vi "отчет по плавке1.vi"(8 "disk":string, 11 "rasp":string[][](array[string])) -> ()   [LabVIEW 2016]
uses:
  Granule-2000AT/PC/llb/Library.lvlib
panel:
  out "P plasmatron":string[](array[string])
  out "P camera":string[](array[string])
  out "PV":string[](array[string])
  out "U_ist":string[](array[string])
  out "I_ist":string[](array[string])
  out "Actual speed":string[](array[string])
  out "Rotation":string[](array[string])
  out "data":string[](array[string])
  out "Mark":string
  out "Billet numer":string caption="Billet\nnumer"
  out "End record":string caption="End of\nrecord"
  out "Start record":string caption="Start\nrecording"
  out "Diametr":string
  in  "Tab Control":T1(tab)
  out "Rotation":cluster{"data dbl":dbl[], dbl[]}(graph)
  out "Actual sped":cluster{"data dbl":dbl[], dbl[]}(graph)
  out "PV зазор":cluster{"data dbl":dbl[], dbl[]}(graph)
  out "I_ист":cluster{"data dbl":dbl[], dbl[]}(graph)
  out "U_ист":cluster{"data dbl":dbl[], dbl[]}(graph)
  out "Presure":cluster{"data dbl":dbl[], dbl[]}[](graph)
  out "Status":u8(slide) scale=0.0..3.0
  in  "Process Stop Button":bool
  in  "Copy Button":bool
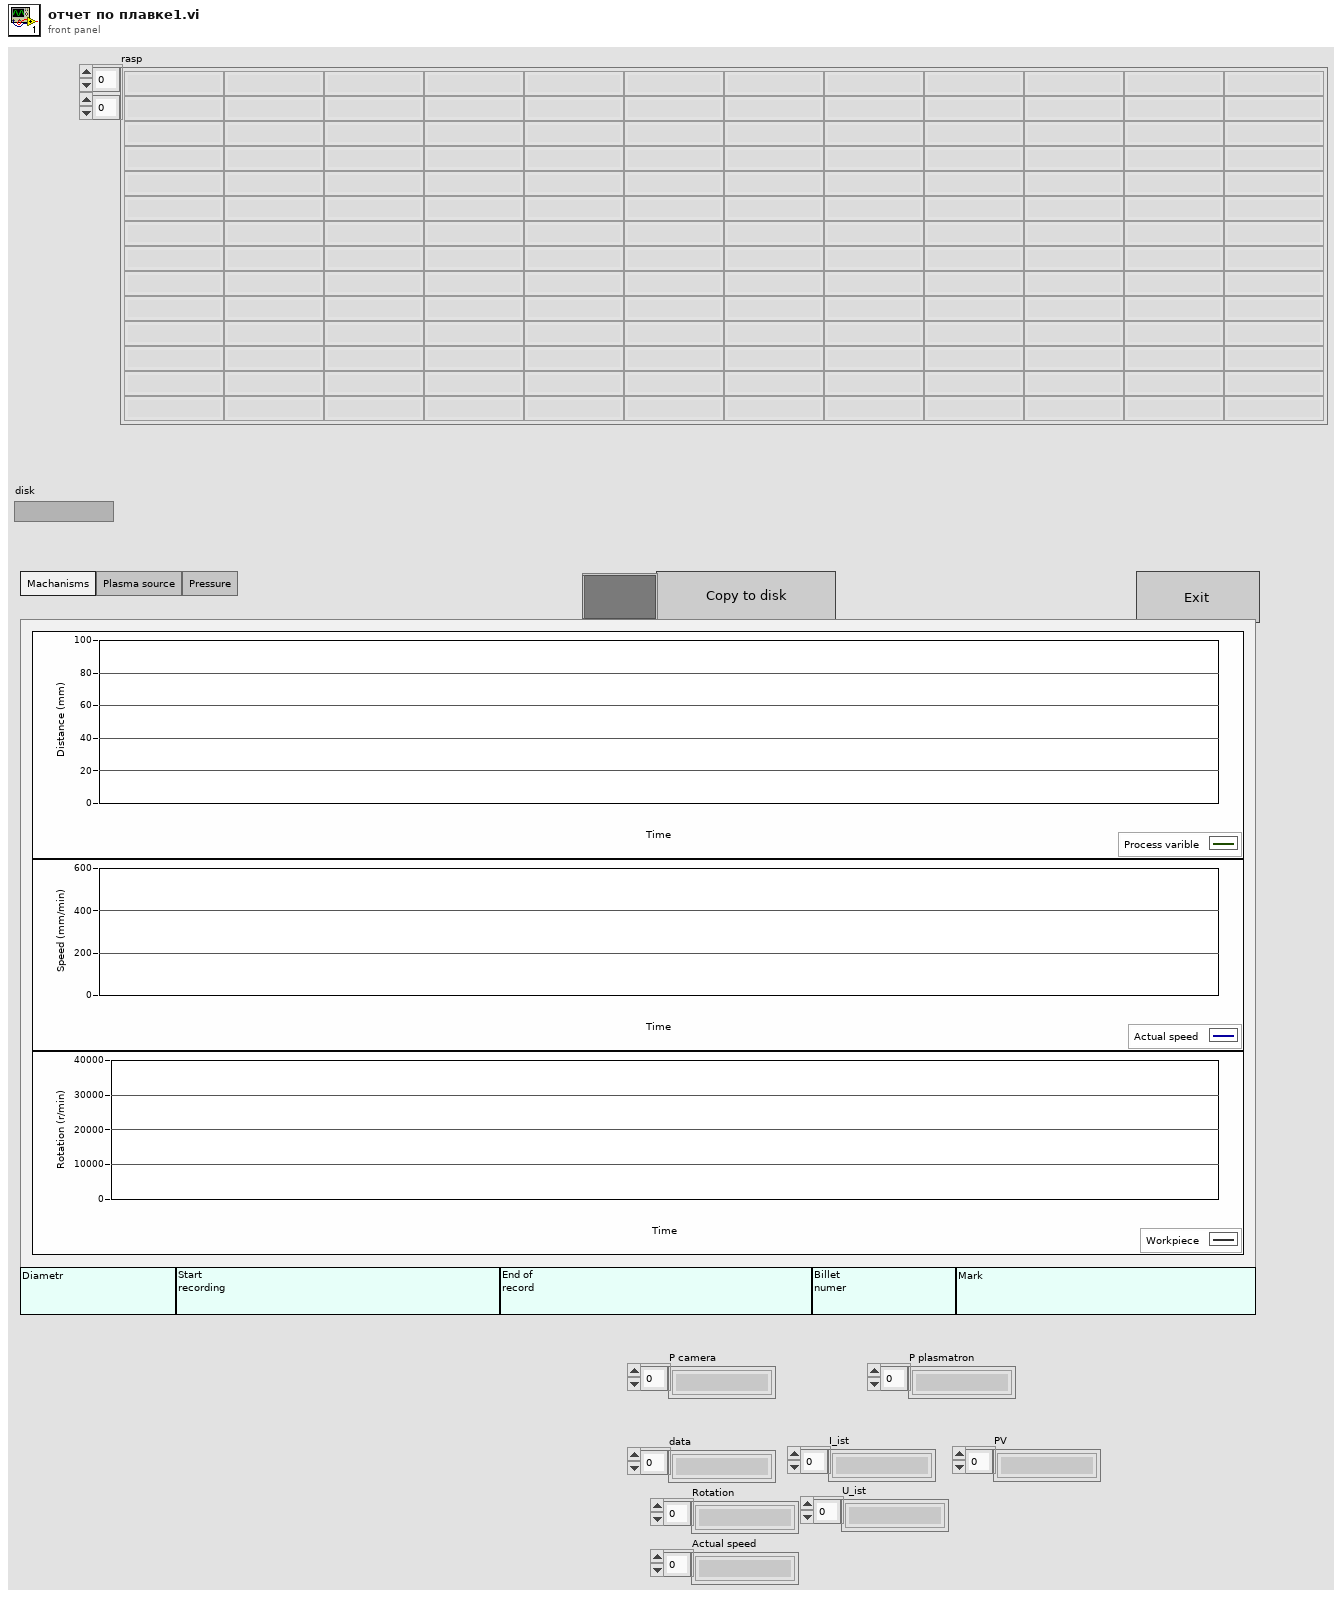
[diagram p1: front panel]
types:
  T1 = enum32{"Machanisms", "Plasma source", "Pressure"}
  T2 = cluster{cluster{"data dbl":dbl[], dbl[]}, cluster{"data dbl":dbl[], dbl[]}, cluster{"data dbl":dbl[], dbl[]}, "String":string, "String":string, "String":string, "String":string, "String":string}
  T3 = cluster{"String":string, "String":string, "String":string, "String":string, "String":string, cluster{"data dbl":dbl[], dbl[]}, cluster{"data dbl":dbl[], dbl[]}, cluster{"data dbl":dbl[], dbl[]}[]}
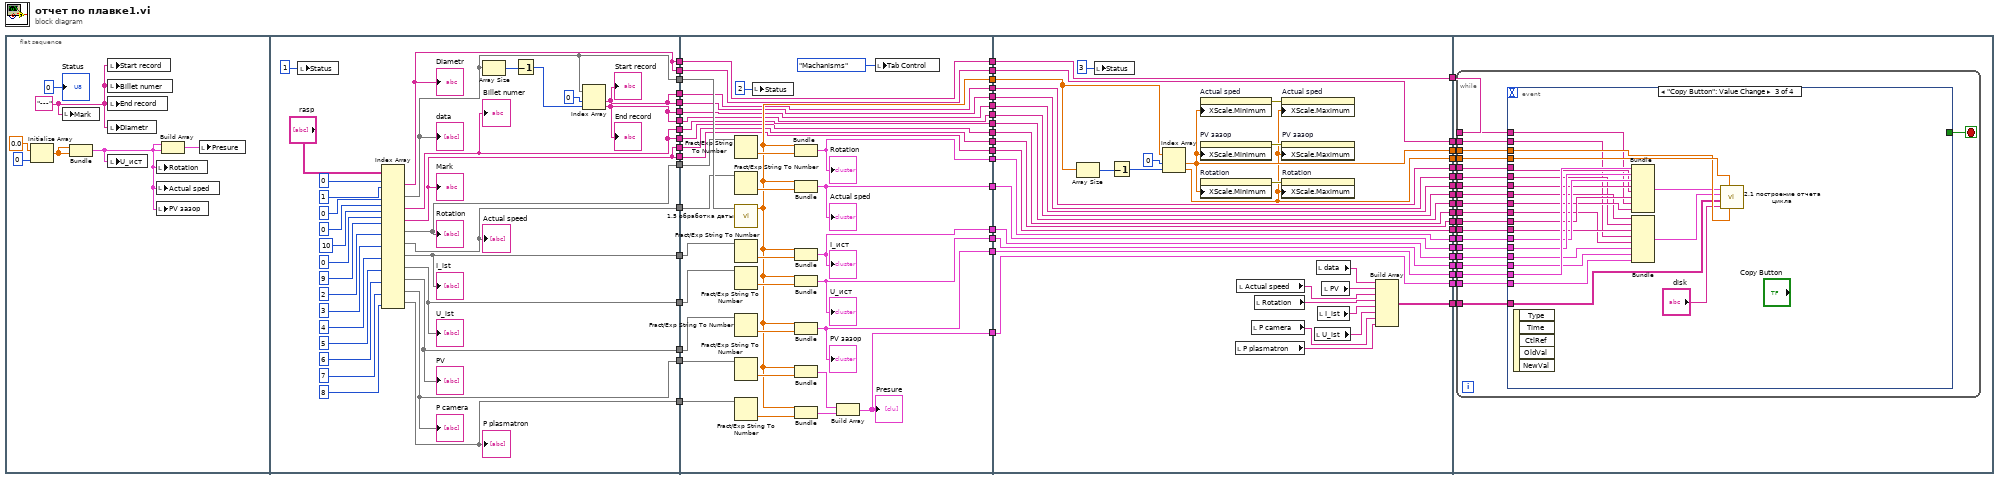
[diagram p0: block diagram]
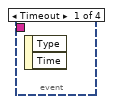
[diagram p2: hidden frame]
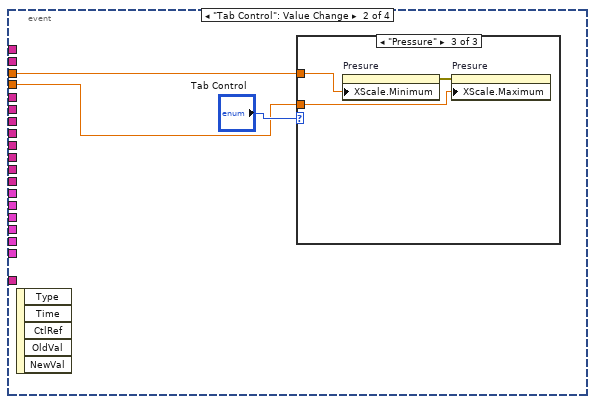
[diagram p3: hidden frame]
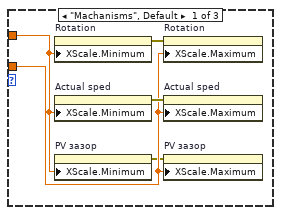
[diagram p4: hidden frame]
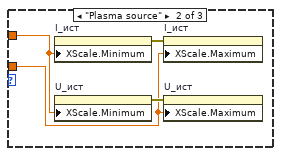
[diagram p5: hidden frame]
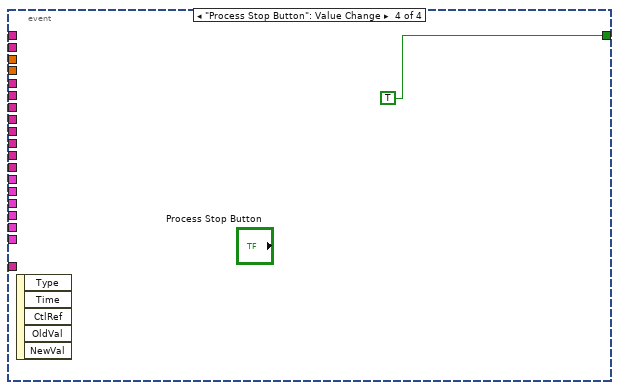
[diagram p6: hidden frame]
diagram:
  n1 = flat-sequence {
    tunnel: [w83] -> w54
    tunnel: [w81] -> w53
    tunnel: [w79] -> w52
    tunnel: [w75] -> w51
    tunnel: [w74] -> w50
    tunnel: [w73] -> w49
    tunnel: [w70] -> w48
    tunnel: [w69] -> w47
    tunnel: [w67] -> w34
    tunnel: [w66] -> w31
    tunnel: [w65] -> w28
    tunnel: [w64] -> w25
    tunnel: [w63] -> w22
    tunnel: [w67] -> w19
    tunnel: [w66] -> w16
    tunnel: [w65] -> w13
    tunnel: [w64] -> w10
    tunnel: [w63] -> w7
    tunnel: w54 -> [w129]
    tunnel: w53 -> [w128]
    tunnel: w52 -> [w126]
    tunnel: w51 -> [w124]
    tunnel: w50 -> [w122]
    tunnel: w49 -> [w119]
    tunnel: w48 -> [w116]
    tunnel: w47 -> [w115]
    tunnel: [w111] -> w46
    tunnel: [w109] -> w41
    tunnel: [w108] -> w39
    tunnel: [w107] -> w37
    tunnel: [w106] -> w35
    tunnel: w34 -> [w106]
    tunnel: [w105] -> w32
    tunnel: w31 -> [w105]
    tunnel: [w104] -> w29
    tunnel: w28 -> [w104]
    tunnel: [w103] -> w26
    tunnel: w25 -> [w103]
    tunnel: [w102] -> w23
    tunnel: w22 -> [w102]
    tunnel: [w101] -> w20
    tunnel: w19 -> [w101]
    tunnel: [w100] -> w17
    tunnel: w16 -> [w100]
    tunnel: [w99] -> w14
    tunnel: w13 -> [w99]
    tunnel: [w98] -> w11
    tunnel: w10 -> [w98]
    tunnel: [w97] -> w8
    tunnel: w7 -> [w97]
    tunnel: [w96] -> w5
    tunnel: [w95] -> w3
    tunnel: [w94] -> w1
    tunnel: w46 -> [w163]
    tunnel: [w157] -> w45
    tunnel: [w156] -> w44
    tunnel: [w146] -> w43
    tunnel: [w145] -> w42
    tunnel: w41 -> [w145]
    tunnel: [w144] -> w40
    tunnel: w39 -> [w144]
    tunnel: [w143] -> w38
    tunnel: w37 -> [w143]
    tunnel: [w142] -> w36
    tunnel: w35 -> [w142]
    tunnel: [w141] -> w33
    tunnel: w32 -> [w141]
    tunnel: [w140] -> w30
    tunnel: w29 -> [w140]
    tunnel: [w139] -> w27
    tunnel: w26 -> [w139]
    tunnel: [w138] -> w24
    tunnel: w23 -> [w138]
    tunnel: [w137] -> w21
    tunnel: w20 -> [w137]
    tunnel: [w136] -> w18
    tunnel: w17 -> [w136]
    tunnel: [w135] -> w15
    tunnel: w14 -> [w135]
    tunnel: [w134] -> w12
    tunnel: w11 -> [w134]
    tunnel: [w133] -> w9
    tunnel: w8 -> [w133]
    tunnel: [w132] -> w6
    tunnel: w5 -> [w132]
    tunnel: [w131] -> w4
    tunnel: w3 -> [w131]
    tunnel: [w130] -> w2
    tunnel: w1 -> [w130]
    tunnel: w45 -> [w183]
    tunnel: w44 -> [w182]
    tunnel: w43 -> [w181]
    tunnel: w42 -> [w180]
    tunnel: w40 -> [w179]
    tunnel: w38 -> [w178]
    tunnel: w36 -> [w177]
    tunnel: w33 -> [w176]
    tunnel: w30 -> [w175]
    tunnel: w27 -> [w174]
    tunnel: w24 -> [w173]
    tunnel: w21 -> [w172]
    tunnel: w18 -> [w171]
    tunnel: w15 -> [w170]
    tunnel: w12 -> [w169]
    tunnel: w9 -> [w168]
    tunnel: w6 -> [w167]
    tunnel: w4 -> [w166]
    tunnel: w2 -> [w165]
    frame #0 {
      w57 = "---" ("Billet numer")
      n2 = Initialize Array(0.0, 0 ("dimension size")) -> (w59:dbl[])
      n3 = local write "Mark"(w57) -> ()
      n4 = Bundle(w59, w59) -> (w56:cluster{dbl[], dbl[]})  [unwired: 1 in]
      n5 = local write "Start record"(w57) -> ()
      n6 = local write "Billet numer"(w57) -> ()
      n7 = local write "End record"(w57) -> ()
      n8 = local write "Diametr"(w57) -> ()
      n9 = local write "U_ист"(w56) -> ()
      n10 = local write "Rotation"(w56) -> ()
      n11 = local write "Actual sped"(w56) -> ()
      n12 = local write "PV зазор"(w56) -> ()
      n13 = Build Array(w56, w56) -> (w55:cluster{dbl[], dbl[]}[])
      n14 = local write "Presure"(w55) -> ()
      "Status" <- u8 0 ("Status")
    }
    frame #1 {
      n15 = local write "Status"(u8 1 ("Status")) -> ()
      n16 = Index Array(array="rasp", index (row) #1=0 ("disabled index (row)"), index (col) #1=1 ("disabled index (col)"), index (col) #2=0 ("index (col)"), index (row) #3=0 ("disabled index (row)"), index (col) #3=10 ("disabled index (col)"), index (row) #4=0 ("disabled index (row)"), index (col) #4=9 ("index (col)"), index (col) #5=2 ("index (col)"), index (col) #6=3 ("index (col)"), index (col) #7=4 ("index (col)"), index (col) #8=5 ("index (col)"), index (col) #9=6 ("index (col)"), index (col) #10=7 ("index (col)"), index (col) #11=8 ("index (col)")) -> (element #1=w64:string, element #2=w83:string[], element #3=w63:string, element #4=w65:string, element #5=w81:string[], element #6=w79:string[], element #7=w74:string[], element #8=w73:string[], element #9=w75:string[], element #10=w70:string[], element #11=w69:string[])  [unwired: 8 in]
      "Diametr" <- w64
      "Billet numer" <- w63
      "Mark" <- w65
      "data" <- w83
      "Rotation" <- w81
      "Actual speed" <- w79
      "I_ist" <- w74
      "U_ist" <- w73
      "PV" <- w75
      "P camera" <- w70
      "P plasmatron" <- w69
      n17 = Array Size(array=w83) -> (size(s)=w90:i32)
      n18 = Decrement(x=w90) -> (x-1=w89:i32)
      n19 = Index Array(array=w83, index #1=0 ("index"), index #2=w89) -> (element #1=w66:string, element #2=w67:string)
      "Start record" <- w66
      "End record" <- w67
    }
    frame #2 {
      n20 = Fract/Exp String To Number(string=w128) -> (number=w127:dbl[])  [unwired: 3 in, 1 out]
      n21 = Fract/Exp String To Number(string=w126) -> (number=w125:dbl[])  [unwired: 3 in, 1 out]
      n22 = call "1.5 обработка даты.vi"("data"=w129) -> ("data dbl"=w111:dbl[])  [unwired: 10 in]
      n23 = Fract/Exp String To Number(string=w122) -> (number=w121:dbl[])  [unwired: 3 in, 1 out]
      n24 = Fract/Exp String To Number(string=w119) -> (number=w120:dbl[])  [unwired: 3 in, 1 out]
      n25 = Fract/Exp String To Number(string=w124) -> (number=w123:dbl[])  [unwired: 3 in, 1 out]
      n26 = Fract/Exp String To Number(string=w116) -> (number=w117:dbl[])  [unwired: 3 in, 1 out]
      n27 = Fract/Exp String To Number(string=w115) -> (number=w118:dbl[])  [unwired: 3 in, 1 out]
      n28 = local write "Status"(u8 2 ("Status")) -> ()
      n29 = Bundle("data dbl"=w111, w127) -> (w107:cluster{"data dbl":dbl[], dbl[]})  [unwired: 1 in]
      "Rotation" <- w107
      n30 = Bundle("data dbl"=w111, w125) -> (w108:cluster{"data dbl":dbl[], dbl[]})  [unwired: 1 in]
      "Actual sped" <- w108
      n31 = Bundle("data dbl"=w111, w121) -> (w96:cluster{"data dbl":dbl[], dbl[]})  [unwired: 1 in]
      "I_ист" <- w96
      n32 = Bundle("data dbl"=w111, w120) -> (w95:cluster{"data dbl":dbl[], dbl[]})  [unwired: 1 in]
      "U_ист" <- w95
      n33 = Bundle("data dbl"=w111, w123) -> (w109:cluster{"data dbl":dbl[], dbl[]})  [unwired: 1 in]
      "PV зазор" <- w109
      n34 = Bundle("data dbl"=w111, w117) -> (w114:cluster{"data dbl":dbl[], dbl[]})  [unwired: 1 in]
      n35 = Bundle("data dbl"=w111, w118) -> (w113:cluster{"data dbl":dbl[], dbl[]})  [unwired: 1 in]
      n36 = Build Array(w114, w113) -> (w94:cluster{"data dbl":dbl[], dbl[]}[])
      "Presure" <- w94
      n37 = local write "Tab Control"(T1."Machanisms" ("Tab Control")) -> ()
    }
    frame #3 {
      n38 = Array Size(array=w163) -> (size(s)=w164:i32)
      n39 = local write "Status"(u8 3 ("Status")) -> ()
      n40 = Decrement(x=w164) -> (x-1=w161:i32)
      n41 = Index Array(array=w163, index #1=0 ("index"), index #2=w161) -> (element #1=w157:dbl, element #2=w156:dbl)
      n42 = property on="Actual sped" class="XYGraph (strict)"("XScale.Minimum"=w157) -> (error out=w159:errorcluster)  [unwired: 2 in, 1 out]
      n43 = property on="PV зазор" class="XYGraph (strict)"("XScale.Minimum"=w157) -> (error out=w158:errorcluster)  [unwired: 2 in, 1 out]
      n44 = property on="Rotation" class="XYGraph (strict)"("XScale.Minimum"=w157) -> (error out=w160:errorcluster)  [unwired: 2 in, 1 out]
      n45 = local read "P plasmatron"() -> (w147:string[])
      n46 = local read "Actual speed"() -> (w152:string[])
      n47 = local read "P camera"() -> (w148:string[])
      n48 = local read "Rotation"() -> (w151:string[])
      n49 = property on="Actual sped" class="XYGraph (strict)"(error in=w159, "XScale.Maximum"=w156) -> ()  [unwired: 1 in, 2 out]
      n50 = property on="PV зазор" class="XYGraph (strict)"(error in=w158, "XScale.Maximum"=w156) -> ()  [unwired: 1 in, 2 out]
      n51 = property on="Rotation" class="XYGraph (strict)"(error in=w160, "XScale.Maximum"=w156) -> ()  [unwired: 1 in, 2 out]
      n52 = local read "U_ist"() -> (w149:string[])
      n53 = local read "data"() -> (w154:string[])
      n54 = local read "I_ist"() -> (w150:string[])
      n55 = local read "PV"() -> (w153:string[])
      n56 = Build Array(w154, w153, w152, w151, w150, w149, w148, w147) -> (w146:string[][])
    }
    frame #4 {
      n57 = while {
        tunnel: w183 -> [w203]
        tunnel: w182 -> [w202]
        tunnel: w181 -> [w200]
        tunnel: w180 -> [w199]
        tunnel: w179 -> [w198]
        tunnel: w178 -> [w197]
        tunnel: w177 -> [w196]
        tunnel: w176 -> [w195]
        tunnel: w175 -> [w194]
        tunnel: w174 -> [w193]
        tunnel: w173 -> [w192]
        tunnel: w172 -> [w191]
        tunnel: w171 -> [w190]
        tunnel: w170 -> [w189]
        tunnel: w169 -> [w188]
        tunnel: w168 -> [w187]
        tunnel: w167 -> [w186]
        tunnel: w166 -> [w185]
        tunnel: w165 -> [w184]
        stop <- w201 stop-if-true
        n58 = event shown="[2] \"Copy Button\": Value Change" {
          selector: _ -> [_ _ _ _]
          dyn-events: _ -> [_ _ _ _]
          timeout: _ -> [_ _ _ _]
          tunnel: w203 -> [_ w205 w239 _]
          tunnel: w202 -> [_ w204 w240 _]
          tunnel: [_ _ _ TRUE] -> w201
          tunnel: w200 -> [_ _ w238 _]
          tunnel: w199 -> [_ _ w236 _]
          tunnel: w198 -> [_ _ w235 _]
          tunnel: w197 -> [_ _ w234 _]
          tunnel: w196 -> [_ _ w233 _]
          tunnel: w195 -> [_ _ w232 _]
          tunnel: w194 -> [_ _ w231 _]
          tunnel: w193 -> [_ _ w230 _]
          tunnel: w192 -> [_ _ w229 _]
          tunnel: w191 -> [_ _ w227 _]
          tunnel: w190 -> [_ _ w226 _]
          tunnel: w189 -> [_ _ w225 _]
          tunnel: w188 -> [_ _ w224 _]
          tunnel: w187 -> [_ _ w223 _]
          tunnel: w186 -> [_ _ w222 _]
          tunnel: w185 -> [_ _ w221 _]
          tunnel: w184 -> [_ _ w220 _]
          event Timeout {
            n59 = event-data() -> ()  [unwired: 1 in, 2 out]
          }
          event "Tab Control": Value Change {
            n60 = event-data() -> ()  [unwired: 1 in, 5 out]
            n61 = case shown="\"Pressure\"" "Tab Control" {
              tunnel: w205 -> [w209 w213 w218]
              tunnel: w204 -> [w208 w212 w217]
              frame "Machanisms", Default {
                n62 = property on="Rotation" class="XYGraph (strict)"("XScale.Minimum"=w209) -> (error out=w211:errorcluster)  [unwired: 2 in, 1 out]
                n63 = property on="Actual sped" class="XYGraph (strict)"("XScale.Minimum"=w209) -> (error out=w210:errorcluster)  [unwired: 2 in, 1 out]
                n64 = property on="PV зазор" class="XYGraph (strict)"("XScale.Minimum"=w209) -> (error out=w207:errorcluster)  [unwired: 2 in, 1 out]
                n65 = property on="Rotation" class="XYGraph (strict)"(error in=w211, "XScale.Maximum"=w208) -> ()  [unwired: 1 in, 2 out]
                n66 = property on="Actual sped" class="XYGraph (strict)"(error in=w210, "XScale.Maximum"=w208) -> ()  [unwired: 1 in, 2 out]
                n67 = property on="PV зазор" class="XYGraph (strict)"(error in=w207, "XScale.Maximum"=w208) -> ()  [unwired: 1 in, 2 out]
              }
              frame "Plasma source" {
                n68 = property on="I_ист" class="XYGraph (strict)"("XScale.Minimum"=w213) -> (error out=w215:errorcluster)  [unwired: 2 in, 1 out]
                n69 = property on="U_ист" class="XYGraph (strict)"("XScale.Minimum"=w213) -> (error out=w214:errorcluster)  [unwired: 2 in, 1 out]
                n70 = property on="I_ист" class="XYGraph (strict)"(error in=w215, "XScale.Maximum"=w212) -> ()  [unwired: 1 in, 2 out]
                n71 = property on="U_ист" class="XYGraph (strict)"(error in=w214, "XScale.Maximum"=w212) -> ()  [unwired: 1 in, 2 out]
              }
              frame "Pressure" {
                n72 = property on="Presure" class="XYGraph (strict)"("XScale.Minimum"=w218) -> (error out=w216:errorcluster)  [unwired: 2 in, 1 out]
                n73 = property on="Presure" class="XYGraph (strict)"(error in=w216, "XScale.Maximum"=w217) -> ()  [unwired: 1 in, 2 out]
              }
            }
          }
          event "Copy Button": Value Change {
            n74 = event-data() -> ()  [unwired: 1 in, 5 out]
            n75 = Bundle(w236, w235, w234, "String"=w233, "String"=w232, "String"=w231, "String"=w230, "String"=w229) -> (w228:T2)  [unwired: 1 in]
            n76 = Bundle("String"=w227, "String"=w226, "String"=w225, "String"=w224, "String"=w223, w222, w221, w220) -> (w219:T3)  [unwired: 1 in]
            n77 = call "2.1 построение отчета цикла.vi"("X Scale.Range:Minimum"=w239, "X Scale.Range:Maximum"=w240, "disk"="disk", "appended array"=w238, "Cluster 2"=w219, "Cluster"=w228) -> ()  [unwired: 6 in]
          }
          event "Process Stop Button": Value Change {
            n78 = event-data() -> ()  [unwired: 1 in, 5 out]
          }
        }
      }
    }
  }
